vi "SAM-Apply.vi"(0 "SAM In":T1, 7 "X":dbl[](array[numeric]), 9 "Sampling Rate (Hz)":dbl, 11 "error in (no error)":errorcluster) -> (4 "SAM Out":T1, 8 "Modulated X":dbl[](array[numeric]), 15 "error out":errorcluster)   [LabVIEW 2020]
uses:
  SAM Params.ctl
  <vilib>/Analysis/NI_AALBase.lvlib
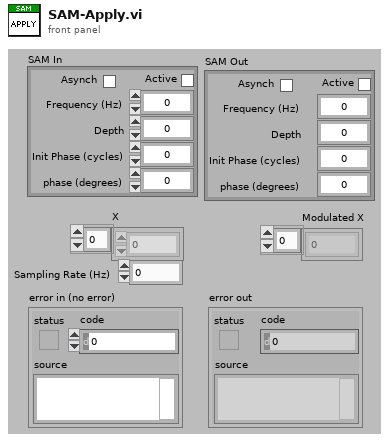
[diagram p1: front panel]
types:
  T1 = typedef "SAM Params.ctl" = cluster{"Active":bool, "Frequency (Hz)":dbl, "Depth":dbl, "Init Phase (cycles)":dbl, "phase (degrees)":dbl, "Asynch":bool}
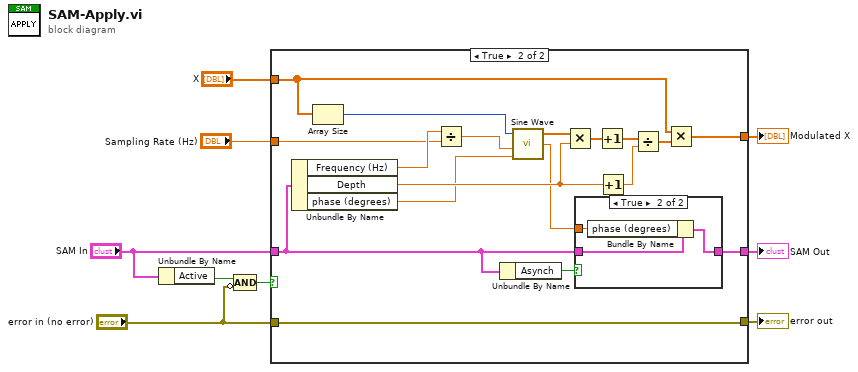
[diagram p0: block diagram]
diagram:
  n1 = Unbundle By Name("SAM In") -> ("Active"=w8:bool)
  n2 = Compound Arithmetic op=AND(w8, invert "error in (no error)") -> (w7:bool)
  n3 = case shown="True" w7 {
    tunnel: [w11 w30] -> w9
    tunnel: "error in (no error)" -> [w11 w30]
    tunnel: "SAM In" -> [w10 w14]
    tunnel: "Sampling Rate (Hz)" -> [_ w20]
    tunnel: "X" -> [w12 w21]
    tunnel: [w12 w15] -> w4
    tunnel: [w10 w17] -> w3
    frame False {
    }
    frame True {
      n4 = Unbundle By Name(w14) -> ("Frequency (Hz)"=w29:dbl, "Depth"=w24:dbl, "phase (degrees)"=w19:dbl)
      n5 = Array Size(array=w21) -> (size(s)=w22:i32)
      n6 = Divide(x=w29, y=w20) -> (x/y=w28:dbl)
      n7 = Unbundle By Name(w14) -> ("Asynch"=w13:bool)
      n8 = call <vilib>:"Sine Wave.vi"("samples"=w22, "frequency"=w28, "phase in"=w19) -> ("sine wave"=w27:dbl[], "phase out"=w18:dbl)  [unwired: 2 in, 1 out]
      n9 = Multiply(x=w27, y=w24) -> (x*y=w26:dbl[])
      n10 = case shown="True" w13 {
        tunnel: w18 -> [_ w34]
        tunnel: [w31 w33] -> w17
        tunnel: w14 -> [w31 w32]
        frame False {
        }
        frame True {
          n11 = Bundle By Name(cluster=w32, "phase (degrees)"=w34) -> (w33:T1)
        }
      }
      n12 = Increment(x=w26) -> (x+1=w25:dbl[])
      n13 = Increment(x=w24) -> (x+1=w23:dbl)
      n14 = Divide(x=w25, y=w23) -> (x/y=w16:dbl[])
      n15 = Multiply(x=w21, y=w16) -> (x*y=w15:dbl[])
    }
  }
  "error out" <- w9
  "Modulated X" <- w4
  "SAM Out" <- w3
